vi "rpr -- get two wings.vi"() -> ()   [LabVIEW 2010]
uses:
  cursor window action.ctl
panel:
  in  "cursor bracket in":refnum<vi>
  out "Plot:   what vs temp 2":cluster{dbl[], dbl[]}[](graph)=[{[50.568, 50.917, 51.261, 51.607, 51.95, 52.297, 52.649, 53.006, 53.352, 53.695, 54.046, 54.395, 54.753, 55.102, 55.455, 55.796, 56.14, 56.492, 56.84, 57.184, 57.526, 57.871, 58.219, 58.576, 58.937, 59.283, 59.623, 59.961, 60.307, 60.656, 61.006, 61.353, 61.697, 62.043, 62.391, 62.735, 63.089, 63.443, 63.783, 64.129, 64.474, 64.819, 65.164, 65.51, 65.863, 66.211, 66.556, 66.904, 67.246, 67.591, 67.932, 68.275, 68.621, 68.966, 69.31, 69.652, 69.995, 70.336, 70.68, 71.03, 71.377, 71.721, 72.065, 72.406, 72.751, 73.094, 73.436, 73.781, 74.123, 74.47, 74.816, 75.164, 75.503, 75.847, 76.183, 76.524, 76.864, 77.206, 77.554, 77.902, 78.241, 78.585, 78.928, 79.269, 79.608, 79.941, 80.277, 80.617, 80.965, 81.311, 81.656, 81.997, 82.34, 82.679, 83.022, 83.363, 83.701, 84.039, 84.378, 84.72, 85.065, 85.409, 85.748, 86.09, 86.429, 86.77, 87.108, 87.451, 87.785, 88.12, 88.461, 88.801, 89.14, 89.482, 89.821, 90.165, 90.506, 90.844, 91.184, 91.524, 91.864, 92.202, 92.541, 92.883, 93.219, 93.555, 93.897, 94.24, 94.58, 94.924, 95.265, 95.606, 95.946, 96.289, 96.626, 96.963, 97.303, 97.639, 97.98, 98.32, 98.657, 98.994, 99.335, 99.677, 100.017, 100.358, 100.695, 101.037, 101.377, 101.716, 102.056, 102.399, 102.738, 103.075, 103.409, 103.714, 104.061, 104.402, 104.738, 105.07, 105.406, 105.743, 106.086, 106.434, 106.769, 107.107, 107.447, 107.788, 108.128, 108.463, 108.804, 109.144, 109.482, 109.822, 110.16, 110.5, 110.837, 111.173, 111.512, 111.854, 112.192, 112.535, 112.869, 113.209, 113.551, 113.886, 114.22, 114.558, 114.898, 115.236, 115.576, 115.913, 116.252, 116.588, 116.926, 117.267, 117.601, 117.941, 118.275, 118.613, 118.952, 119.294, 119.632, 119.969, 120.303, 120.639, 120.975, 121.311, 121.648, 121.985, 122.321, 122.658, 122.997, 123.335, 123.674, 124.012, 124.348, 124.686, 125.023, 125.36, 125.694, 126.036, 126.373, 126.709, 127.046, 127.382, 127.722, 128.062, 128.4, 128.738, 129.066, 129.397, 129.74, 130.077, 130.411, 130.746, 131.087, 131.425, 131.757, 132.093, 132.423, 132.754, 133.081, 133.403, 133.725, 134.042, 134.359, 134.667, 134.986, 135.381, 135.701, 136.02, 136.328, 136.625, 136.918], [0.48238111111111104, 0.48609111111111114, 0.44962111111111114, 0.4878311111111111, 0.4939511111111111, 0.4796111111111111, 0.4859811111111111, 0.49955111111111106, 0.531631111111111, 0.5312211111111111, 0.5094311111111111, 0.5354511111111111, 0.5416211111111111, 0.5303611111111111, 0.519291111111111, 0.5349311111111111, 0.5236411111111111, 0.555661111111111, 0.5484711111111111, 0.581081111111111, 0.5926811111111111, 0.5866611111111111, 0.599721111111111, 0.544831111111111, 0.5413111111111111, 0.6067811111111111, 0.5752111111111111, 0.699381111111111, 0.5701811111111111, 0.5595211111111111, 0.6914411111111111, 0.612281111111111, 0.7042711111111111, 0.6801611111111111, 0.8049011111111111, 0.7785711111111111, 0.7562811111111111, 0.8775911111111111, 0.6216811111111111, 0.4662211111111111, 0.39060111111111107, 0.35540111111111106, 0.3376611111111111, 0.2965211111111111, 0.20450111111111108, -0.01088888888888892, 0.1271411111111111, 0.12296111111111109, 0.1499011111111111, -0.0389288888888889, 0.019671111111111098, -0.012378888888888911, -0.07840888888888892, -0.1442388888888889, -0.20322888888888893, -0.19372888888888892, -0.17868888888888892, -0.14193888888888892, -0.1596188888888889, -0.03765888888888891, -0.28303888888888895, -0.23724888888888893, -0.2220588888888889, -0.3366988888888889, -0.37551888888888896, -0.3045188888888889, -0.31216888888888894, -0.2778588888888889, -0.30645888888888895, -0.27690888888888887, -0.3512788888888889, -0.34904888888888896, -0.34033888888888886, -0.4198088888888889, -0.45179888888888897, -0.4417588888888889, -0.4199988888888889, -0.4567388888888889, -0.4566188888888889, -0.4698188888888889, -0.48351888888888894, -0.4450088888888889, -0.4343688888888889, -0.47826888888888897, -0.47109888888888896, -0.4693788888888889, -0.45333888888888896, -0.4567888888888889, -0.4531588888888889, -0.450968888888889, -0.44623888888888896, -0.4609888888888889, -0.44589888888888896, -0.46680888888888894, -0.44618888888888897, -0.44721888888888894, -0.4465188888888889, -0.42774888888888896, -0.4246588888888889, -0.43613888888888896, -0.422888888888889, -0.4334888888888889, -0.5087288888888889, -0.3843588888888889, -0.384588888888889, -0.37024888888888896, -0.3322788888888889, -0.3667288888888889, -0.37993888888888894, -0.35333888888888887, -0.3072688888888889, -0.31677888888888894, -0.2908588888888889, -0.2871988888888889, -0.28927888888888886, -0.2754388888888889, -0.2538688888888889, -0.2713388888888889, -0.2504288888888889, -0.2402188888888889, -0.23412888888888891, -0.23181888888888894, -0.2447588888888889, -0.2397188888888889, -0.2292988888888889, -0.23631888888888888, -0.24041888888888893, -0.2335488888888889, -0.2246188888888889, -0.22349888888888889, -0.2160788888888889, -0.21464888888888892, -0.2277988888888889, -0.22914888888888893, -0.2365988888888889, -0.2300588888888889, -0.2212288888888889, -0.2178088888888889, -0.2281088888888889, -0.22291888888888892, -0.28493888888888896, -0.2380488888888889, -0.22785888888888892, -0.24313888888888893, -0.2302188888888889, -0.23642888888888888, -0.2598288888888889, -0.26863888888888887, -0.26024888888888886, -0.2716788888888889, -0.25154888888888893, -0.2569288888888889, -0.2620688888888889, -0.2701888888888889, -0.2481088888888889, -0.2806388888888889, -0.2588988888888889, -0.33175888888888894, -0.33177888888888896, -0.32653888888888893, -0.3356688888888889, -0.30977888888888894, -0.2955388888888889, -0.28283888888888886, -0.26610888888888895, -0.27154888888888895, -0.2507988888888889, -0.2518788888888889, -0.25078888888888895, -0.23685888888888892, -0.23834888888888892, -0.2295188888888889, -0.2326788888888889, -0.2189688888888889, -0.21031888888888892, -0.20272888888888893, -0.1876988888888889, -0.2036288888888889, -0.17873888888888892, -0.1388788888888889, -0.1668388888888889, -0.15771888888888894, -0.14938888888888893, -0.1615688888888889, -0.14716888888888893, -0.1345388888888889, -0.13673888888888888, -0.1449188888888889, -0.14294888888888893, -0.15399888888888894, -0.16492888888888893, -0.1584488888888889, -0.1654988888888889, -0.1617288888888889, -0.1722688888888889, -0.16837888888888888, -0.17185888888888892, -0.20267888888888894, -0.15475888888888892, -0.1702388888888889, -0.15692888888888892, -0.16548888888888894, -0.1584088888888889, -0.16502888888888892, -0.1495888888888889, -0.15055888888888888, -0.15431888888888892, -0.14444888888888893, -0.1469788888888889, -0.13954888888888892, -0.1449588888888889, -0.14570888888888892, -0.1515288888888889, -0.1425388888888889, -0.12855888888888892, -0.14149888888888892, -0.13856888888888894, -0.13368888888888888, -0.1384788888888889, -0.14337888888888892, -0.1491288888888889, -0.14926888888888892, -0.13782888888888892, -0.1521188888888889, -0.1506788888888889, -0.16025888888888892, -0.16059888888888893, -0.15409888888888892, -0.14809888888888892, -0.1461388888888889, -0.1345288888888889, -0.1312088888888889, -0.1359688888888889, -0.09027888888888891, -0.08645888888888892, -0.0857788888888889, -0.08680888888888891, -0.07471888888888892, -0.08092888888888891, -0.08032888888888892, -0.0818288888888889, -0.0915188888888889, -0.09258888888888891, -0.09095888888888892, -0.0976288888888889, -0.09267888888888892, -0.09161888888888892, -0.0887988888888889, -0.0916588888888889, -0.09480888888888891, -0.09968888888888891, -0.09869888888888892, -0.10298888888888891, -0.1084188888888889, -0.10921888888888892]}]
  out "best fit parameters right":dbl[](array[numeric])
  out "best fit parameters left":dbl[](array[numeric])
  in  "gap":dbl
  out "residue right":dbl
  out "residue left":dbl
  out "x-y":dbl[](array[numeric])
  in  "temperature points OUT":dbl[](array[numeric])
  in  "what points out":dbl[](array[numeric])
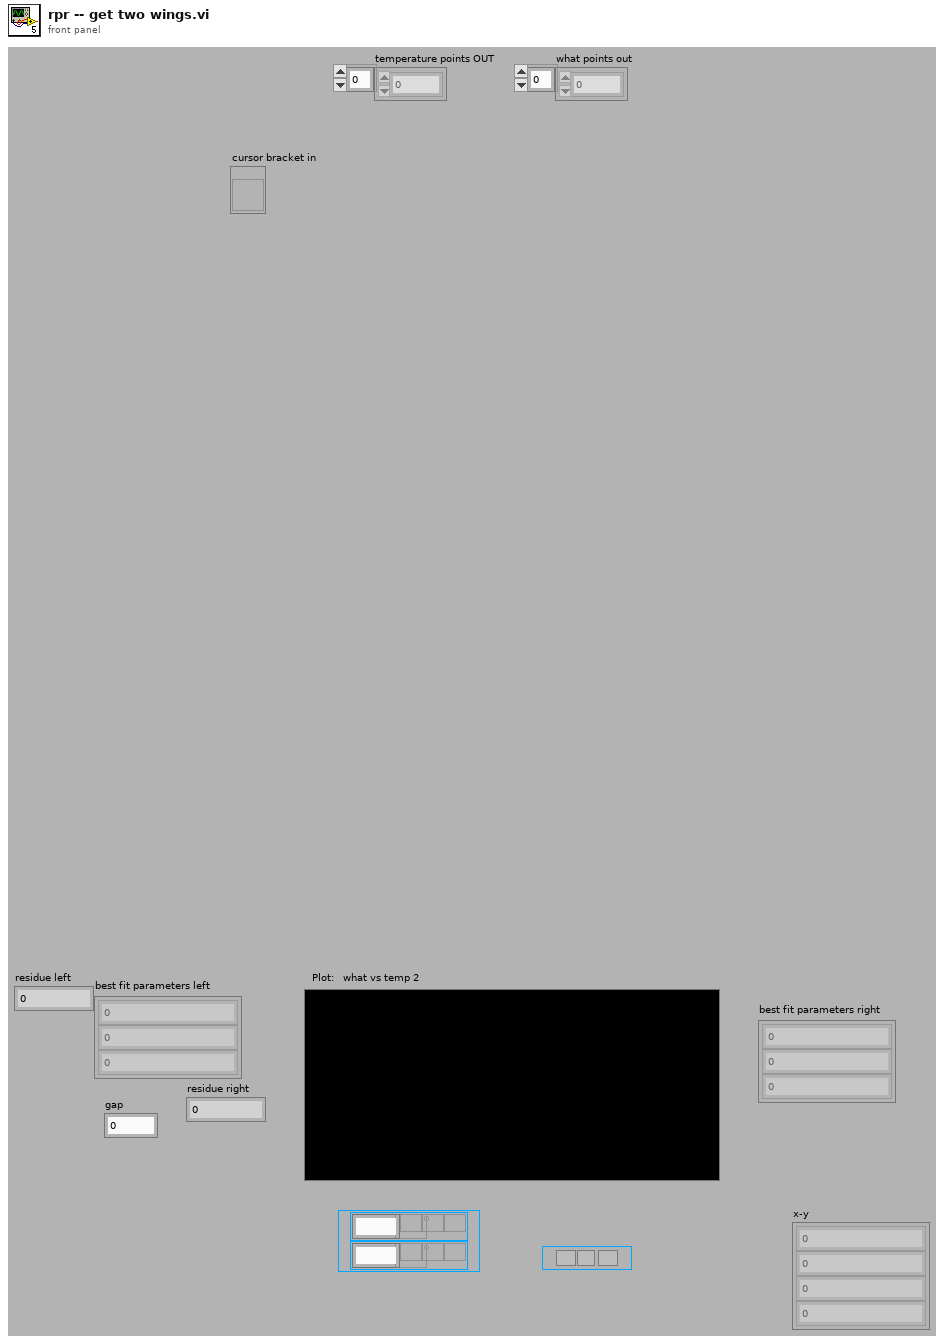
[diagram p1: front panel]
types:
  T1 = typedef "cursor window action.ctl" = enum16{"balance", "h. offset change", "cursor moves", "center change", "window change", "init", "check", "reset", "set y to middle"}
  T2 = typedef "cursor winow.ctl" = cluster{"left":dbl, "right ":dbl, "center":dbl, "window":dbl, "cursors":i32[], "relative":i32, "absolute":i32, "plot ref":refnum<vi>, "Cursor List":T3, "fixed vertical offset":dbl, "vertical offset":dbl, "horizontal offset":dbl, "default window frac":dbl, "kind":enum16{"symmetric", "skewed", "fancy"}}
  T3 = typedef "LVCursorListTypeDef.ctl" = cluster{"Name":string, "Color":u32, "Style":u8, "Point Style":u8, "Name Visible":bool, "Allow Drag":bool, "Cursor Mode":u32, "Plot":i32, "Index":i32, "Position":cluster{"X":dbl, "Y":dbl}, "X Scale":u32, "Y Scale":u32, "Watch Plots":i32[], "Watch All Plots":bool, "Plot Area":i32, "Label Offset":cluster{"X":dbl, "Y":dbl}}[]
  T4 = cluster{"temperature points OUT":dbl[], "what points out":dbl[]}
  T5 = cluster{"temperature points OUT":dbl[], "what points out":dbl[]}[]
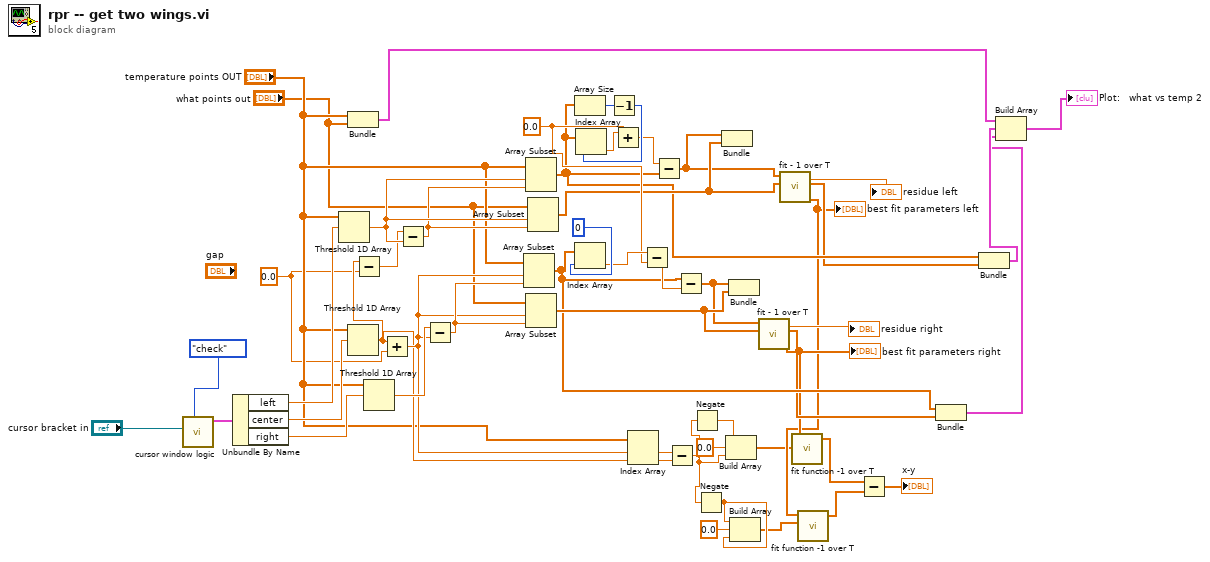
[diagram p0: block diagram]
diagram:
  w1 = 0.0
  w36 = 0.0 ("y")
  n1 = call "cursor window logic.vi"("cursor window action"=cursor_window_action."check", "cursor bracket in"="cursor bracket in") -> ("cursor window out"=w51:T2)  [unwired: 8 in, 1 out]
  n2 = Unbundle By Name(w51) -> ("left"=w49:dbl, "center"=w48:dbl, "right"=w47:dbl)
  n3 = Threshold 1D Array(2:w49, 3:"temperature points OUT") -> (0:w46:dbl)  [unwired: 1 in]
  n4 = Bundle("temperature points OUT"="temperature points OUT", "what points out"="what points out") -> (w31:T4)  [unwired: 1 in]
  n5 = Threshold 1D Array(2:w48, 3:"temperature points OUT") -> (0:w17:dbl)  [unwired: 1 in]
  n6 = Subtract(x=w17, y=w1) -> (x-y=w22:dbl)
  n7 = Threshold 1D Array(2:w47, 3:"temperature points OUT") -> (0:w43:dbl)  [unwired: 1 in]
  n8 = Add(x=w17, y=w1) -> (x+y=w18:dbl)
  n9 = Subtract(x=w22, y=w46) -> (x-y=w45:dbl)
  n10 = Subtract(x=w43, y=w18) -> (x-y=w44:dbl)
  n11 = Array Subset(array="temperature points OUT", index=w18, length=w44) -> (w30:dbl[])
  n12 = Array Subset(array="temperature points OUT", index=w46, length=w45) -> (w29:dbl[])
  n13 = Array Subset(array="what points out", index=w18, length=w44) -> (w33:dbl[])
  n14 = Array Subset(array="what points out", index=w46, length=w45) -> (w34:dbl[])
  n15 = Array Size(array=w29) -> (size(s)=w42:i32)
  n16 = Index Array(array=w30, index=0) -> (element=w37:dbl)
  n17 = Decrement(x=w42) -> (x-1=w41:i32)
  n18 = Index Array(array=w29, index=w41) -> (element=w40:dbl)
  n19 = Add(x=w40, y=w36) -> (x+y=w39:dbl)
  n20 = Index Array(array="temperature points OUT", index #1=w18, index #2=w17) -> (element #1=w16:dbl, element #2=w15:dbl)
  n21 = Subtract(x=w37, y=w36) -> (x-y=w35:dbl)
  n22 = Subtract(x=w39, y=w29) -> (x-y=w23:dbl[])
  n23 = Subtract(x=w16, y=w15) -> (x-y=w10:dbl)
  n24 = Subtract(x=w30, y=w35) -> (x-y=w24:dbl[])
  n25 = Negate(x=w10) -> (-x=w14:dbl)
  n26 = Negate(x=w10) -> (-x=w9:dbl)
  n27 = Bundle(w23, w34) -> ()  [unwired: 1 in, 1 out]
  n28 = Build Array(w14, 0.0 ("y"), w10) -> (w12:dbl[])
  n29 = Bundle(w24, w33) -> ()  [unwired: 1 in, 1 out]
  n30 = Build Array(w9, 0.0 ("y"), w9) -> (w8:dbl[])
  n31 = call "fit - 1 over T.vi"("what points"=w33, "temperature points"=w24) -> ("best fit parameters"=w19:dbl[], "what points out"=w26:dbl[], "residue"=→"residue right":dbl)  [unwired: 5 in, 2 out]
  "best fit parameters right" <- w19
  n32 = call "fit - 1 over T.vi"("what points"=w34, "temperature points"=w23) -> ("best fit parameters"=w13:dbl[], "what points out"=w25:dbl[], "residue"=→"residue left":dbl)  [unwired: 5 in, 2 out]
  "best fit parameters left" <- w13
  n33 = call "fit function -1 over T.vi"("X"=w12, "a"=w19) -> ("f(X,a)"=w7:dbl[])  [unwired: 2 in, 2 out]
  n34 = call "fit function -1 over T.vi"("X"=w8, "a"=w13) -> ("f(X,a)"=w6:dbl[])  [unwired: 2 in, 2 out]
  n35 = Subtract(x=w7, y=w6) -> (x-y=→"x-y":dbl[])
  n36 = Bundle(w30, "what points out"=w26) -> (w27:cluster{dbl[], "what points out":dbl[]})  [unwired: 1 in]
  n37 = Bundle(w29, "what points out"=w25) -> (w28:cluster{dbl[], "what points out":dbl[]})  [unwired: 1 in]
  n38 = Build Array(w31, w28, w27) -> (→"Plot:   what vs temp 2":T5)
